vi "SCT Filter Feature Packs.vi"(7 "Allow or disallow?":enum16{"Allow", "Disallow"}(ring), 9 "localized names":string[](array[string]), 10 "internal names":string[](array[string]), 11 "Feature Packs to filter":string[](array[string])) -> (1 "filtered localized names":string[](array[string]), 2 "filtered internal names":string[](array[string]))   [LabVIEW 2016]
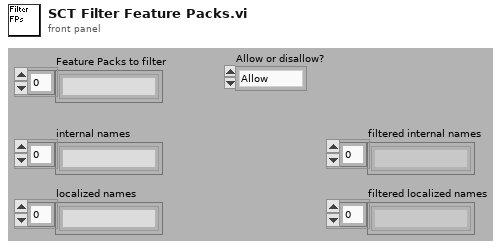
[diagram p1: front panel]
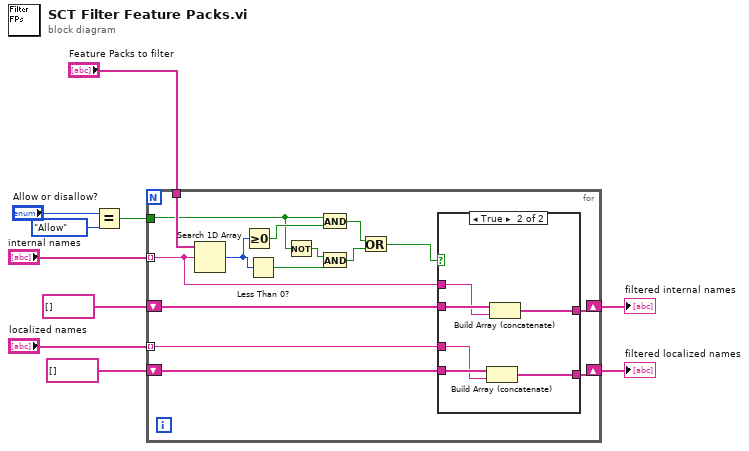
[diagram p0: block diagram]
diagram:
  n1 = Equal?(x="Allow or disallow?", y=enum16{"Allow", "Disallow"}."Allow") -> (x = y?=w1:bool)
  n2 = for {
    tunnel: "internal names" -> [w24] mode=indexing
    tunnel: "localized names" -> [w23] mode=indexing
    shift-right: [w19] -> w10
    shift-left: string[] [] -> [w22]
    shift-right: [w20] -> w9
    shift-left: string[] [] -> [w21]
    tunnel: "Feature Packs to filter" -> [w25]
    tunnel: w1 -> [w14]
    n3 = Search 1D Array(1D array=w25, element=w24) -> (index of element=w13:i32)  [unwired: 1 in]
    n4 = Greater Or Equal To 0?(x=w13) -> (x >= 0?=w16:bool)
    n5 = Less Than 0?(x=w13) -> (x < 0?=w12:bool)
    n6 = Not(x=w14) -> (.not. x?=w15:bool)
    n7 = And(x=w14, y=w16) -> (x .and. y?=w18:bool)
    n8 = And(x=w15, y=w12) -> (x .and. y?=w17:bool)
    n9 = Or(x=w18, y=w17) -> (x .or. y?=w11:bool)
    n10 = case shown="True" w11 {
      tunnel: w24 -> [_ w30]
      tunnel: w23 -> [_ w31]
      tunnel: w22 -> [w27 w33]
      tunnel: w21 -> [w26 w32]
      tunnel: [w26 w29] -> w20
      tunnel: [w27 w28] -> w19
      frame False {
        # "If it's not in the allowed\nlist, filter it out."
      }
      frame True {
        n11 = Build Array (concatenate)(w32, w31) -> (w29:string[])
        n12 = Build Array (concatenate)(w33, w30) -> (w28:string[])
      }
    }
  }
  "filtered internal names" <- w10
  "filtered localized names" <- w9
